vi "Read HW Angle 0 Trim Performed.vi"(6 "error in":errorcluster, 9 "Channel in":u16) -> (0 "error out":errorcluster, 1 "Messages":T1(array[cluster]), 2 "Pass":bool, 3 "Channel out":u16)   [LabVIEW 2023]
uses:
  7ad73885-74d4-4865-958d-ac69876d8a76.vi
  Communication/PCAN2023/PCAN API.lvlib
panel:
  out "Numeric":i32
  in  "stop 1":bool
  out "MessageBuffer out":T2 {"ID" format="%.0x"; "DATA[0]" format="%.0x"; "DATA[1]" format="%.0x"; "DATA[2]" format="%.0x"; "DATA[3]" format="%.0x"; "DATA[4]" format="%.0x"; "DATA[5]" format="%.0x"; "DATA[6]" format="%.0x"; "DATA[7]" format="%.0x"}
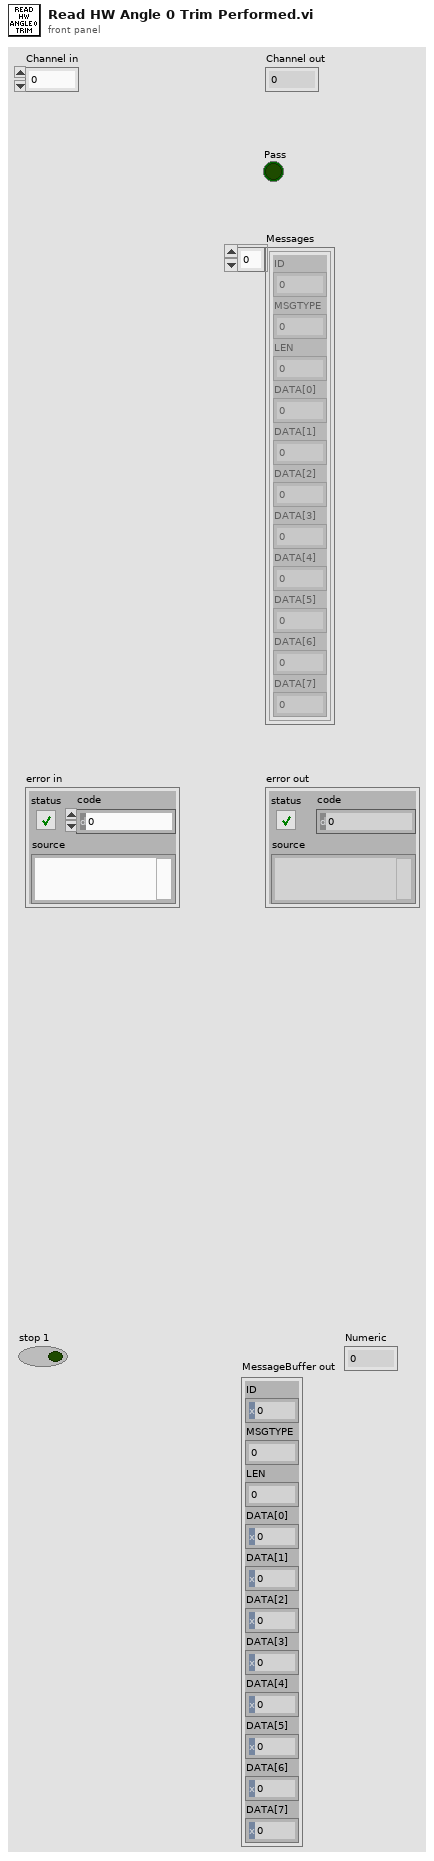
[diagram p1: front panel]
types:
  T1 = cluster{"ID":u32, "MSGTYPE":u8, "LEN":u8, "DATA[0]":u8, "DATA[1]":u8, "DATA[2]":u8, "DATA[3]":u8, "DATA[4]":u8, "DATA[5]":u8, "DATA[6]":u8, "DATA[7]":u8}[]
  T2 = cluster{"ID":u32, "MSGTYPE":u8, "LEN":u8, "DATA[0]":u8, "DATA[1]":u8, "DATA[2]":u8, "DATA[3]":u8, "DATA[4]":u8, "DATA[5]":u8, "DATA[6]":u8, "DATA[7]":u8}
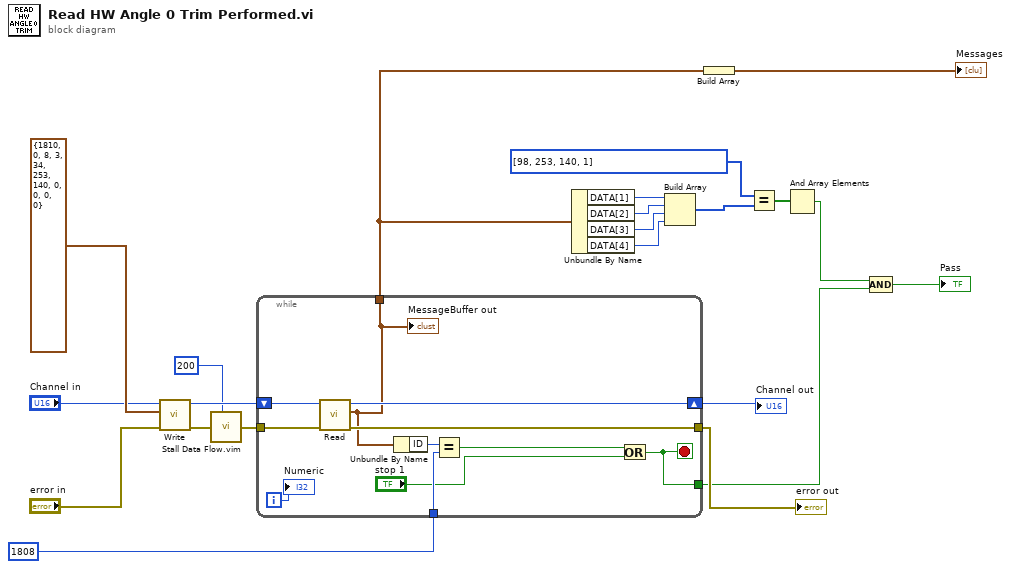
[diagram p0: block diagram]
diagram:
  n1 = call "Write.vi"("error in"="error in", "MessageBuffer"=T2 {"ID"=1810, "MSGTYPE"=0, "LEN"=8, "DATA[0]"=3, "DATA[1]"=34, "DATA[2]"=253, "DATA[3]"=140, "DATA[4]"=0, "DATA[5]"=0, "DATA[6]"=0, "DATA[7]"=0}, "Channel"="Channel in") -> ("error out"=w21:errorcluster, "Channel out"=w20:u16)  [unwired: 5 in, 2 out]
  n2 = call "Stall Data Flow.vim"("value in"=w21, "milliseconds to wait"=u32 200) -> ("value out"=w11:errorcluster)  [unwired: 1 out]
  n3 = while {
    shift-right: [w31] -> w16
    shift-left: w20 -> [w32]
    tunnel: u32 1808 ("ID") -> [w28]
    tunnel: [w24] -> w9
    tunnel: [w25] -> w13
    tunnel: w11 -> [w33]
    tunnel: [w30] -> w15
    i -> [w27]
    stop <- w25 stop-if-true
    n4 = call "Read.vi"("error in"=w33, "Channel"=w32) -> ("error out"=w30:errorcluster, "MessageBuffer out"=w24:T2, "Channel out"=w31:u16)  [unwired: 6 in, 1 out]
    "MessageBuffer out" <- w24
    n5 = Unbundle By Name(w24) -> ("ID"=w29:u32)
    n6 = Equal?(x=w29, y=w28) -> (x = y?=w23:bool)
    n7 = Or(x=w23, y="stop 1") -> (x .or. y?=w25:bool)
    "Numeric" <- w27
  }
  "error out" <- w15
  "Channel out" <- w16
  n8 = Unbundle By Name(w9) -> ("DATA[1]"=w7:u8, "DATA[2]"=w6:u8, "DATA[3]"=w5:u8, "DATA[4]"=w4:u8)
  n9 = Build Array(w7, w6, w5, w4) -> (w3:u8[])
  n10 = Build Array(w9) -> (→"Messages":T1)
  n11 = Equal?(x=u8[] [98, 253, 140, 1], y=w3) -> (x = y?=w2:bool[])
  n12 = And Array Elements(Boolean array=w2) -> (logical AND=w1:bool)
  n13 = Compound Arithmetic op=AND(w1, w13) -> (→"Pass":bool)
